vi "GT Set Adc Config.vi"(8 "error in (no error)":errorcluster caption="错误输入（无错误）", 9 "pAdc":T1, 10 "adc":i16, 11 "cardNum":i16) -> (0 "error out":errorcluster caption="错误输出", 1 "pAdc out":T1, 3 "function return":i16)   [LabVIEW 2014, in "gts.lvlib"]
doc: "GT_API GT_SetAdcConfig(short cardNum,short adc,TAdcConfig *pAdc);"
uses:
  gts.lvlib
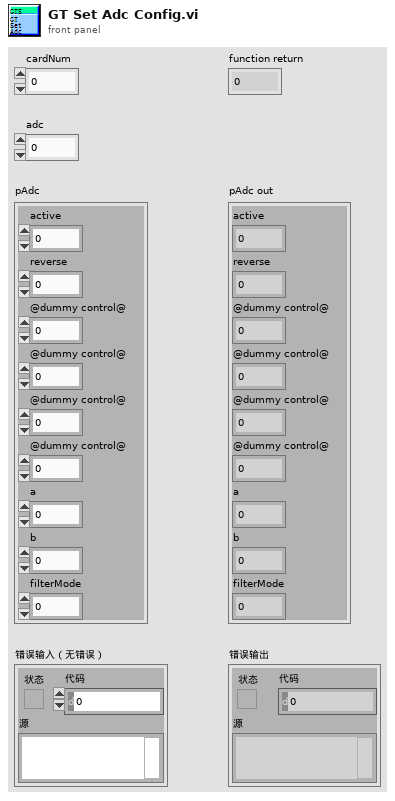
[diagram p1: front panel]
types:
  T1 = cluster{"active":i16, "reverse":i16, "@dummy control@":i8, "@dummy control@":i8, "@dummy control@":i8, "@dummy control@":i8, "a":dbl, "b":dbl, "filterMode":i16}
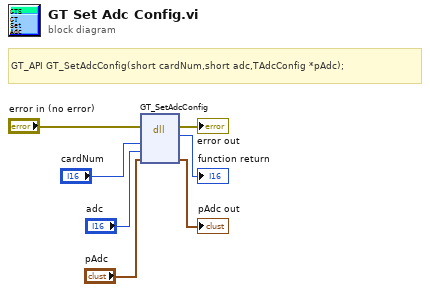
[diagram p0: block diagram]
diagram:
  # "GT_API GT_SetAdcConfig(short cardNum,short adc,TAdcConfig *pAdc);"
  n1 = dll-call lib="PTH2habs D固高科技资料GTS控制卡GTS卡18年上半年资料dllVC32bit\nmulti_cardgts.*" fn="GT_SetAdcConfig"(error in="error in (no error)", "cardNum"="cardNum", "adc"="adc", "pAdc"="pAdc") -> (error out=→"error out":errorcluster, →"function return":i16, "pAdc"=→"pAdc out":T1)  [unwired: 4 in, 1 out]
